vi "Write Element.vi"(8 "error in (no error)":errorcluster, 10 "Element.lvclass":refnum<class "Element.lvclass">, 11 "ParseGDSII in":refnum<class "ParseGDSII.lvclass">) -> (0 "error out":errorcluster, 3 "ParseGDSII out":refnum<class "ParseGDSII.lvclass">)   [LabVIEW 2019]
uses:
  ParseGDSII.lvclass
  Elements/Element.lvclass
  ParseGDSII.lvclass/ParseGDSII.ctl
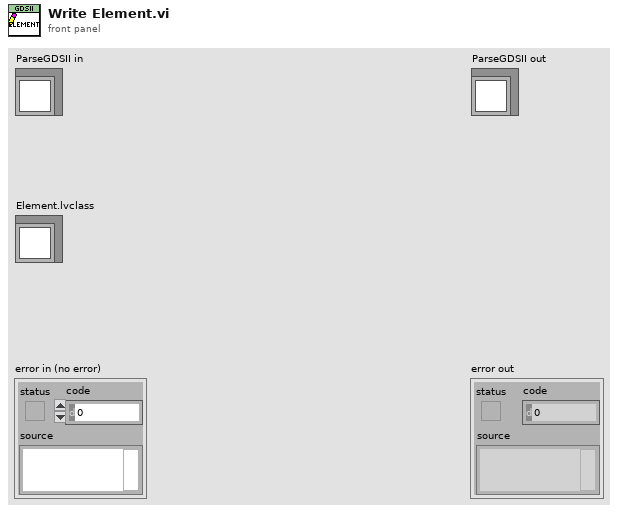
[diagram p1: front panel]
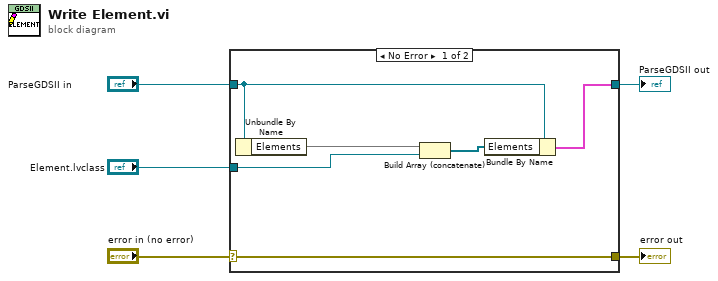
[diagram p0: block diagram]
diagram:
  n1 = case shown="No Error" "error in (no error)" {
    selector: "error in (no error)" -> [w11 w12]
    tunnel: [w11 w12] -> w4
    tunnel: [w10 w13] -> w2
    tunnel: "ParseGDSII in" -> [w9 w13]
    tunnel: "Element.lvclass" -> [w6 _]
    frame No Error {
      n2 = Unbundle By Name(w9) -> ("Elements"=w8)
      n3 = Build Array (concatenate)(w8, w6) -> (w7:refnum<class "Element.lvclass">[])
      n4 = Bundle By Name(cluster=w9, "Elements"=w7) -> (w10:cluster{})
    }
    frame Error {
    }
  }
  "error out" <- w4
  "ParseGDSII out" <- w2
